vi "Measurement UI.vi"() -> ()   [LabVIEW 2025, in "CAN-LIN Frame Generator UI.lvlib"]
uses:
  CAN-LIN Frame Generator UI.lvlib
  Toggle.ctl
  <vilib>/xnet/xnet.llb/XNET Frame Type CAN.ctl
  OOB gRPC Client/RPC Messages/hwval_GenericRequest.ctl
  OOB gRPC Client/RPC Messages/hwval_BoolRequest.ctl
  <vilib>/Utility/sysdir.llb/System Directory Type.ctl
  OOB gRPC Client/OOB gRPC Client.lvlib
panel:
  in  "HELP":bool
  out "cfg err":bool
  in  "PauseResume":bool caption="Pause"
  out "OOB gRPC Port":i32
  in  "Network":string
  in  "LIN interface":string
  in  "CAN interface":string
  in  "SETTINGS":enum32{"CAN", "LIN"}(tab)
  out "Status CAN":string
  in  "Payload CAN":u32[](array[numeric])=[0, 0, 0, 0, 0, 0, 0, 0, 0, 0, 0, 0, 0, 0, 0, 0, 0, 0, 0, 0, 0, 0, 0, 0, 0, 0, 0, 0, 0, 0, 0, 0, 0, 0, 0, 0, 0, 0, 0, 0, 0, 0, 0, 0, 0, 0, 0, 0, 0, 0, 0, 0, 0, 0, 0, 0, 0, 0, 0, 0, 0, 0, 0, 0] format="%x"
  in  "SEND CAN":bool
  in  "DLC CAN":u32=8
  in  "Type CAN":T1 items=["CAN Data"=0, "CAN Remote"=1, "CAN Bus Error"=2, "CAN 2.0 Data"=8, "CAN FD Data"=16, "CAN FD+BRS Data"=24, "J1939 Data"=192, "Delay"=224, "Log Trigger"=225, "Start Trigger"=226]
  in  "ID CAN":u32 format="%x"
  in  "IO Mode CAN":enum32{"CAN", "CAN FD", "CAN FD + BRS"}(ring)
  in  "FD ISO Mode CAN":enum32{"ISO", "Legacy ISO", "Non-ISO"}(ring)
  in  "Baudrate CAN":u32=125000
  in  "FD Baudrate CAN":u32=1000000
  in  "Termination CAN":T2
  in  "INTERFACE NAME CAN":refnum<k21>
  out "Status LIN":string
  in  "Payload LIN":u32[](array[numeric])=[0, 0, 0, 0, 0, 0, 0, 0] format="%x"
  in  "SEND LIN":bool
  in  "DLC LIN":u32=8
  in  "ID LIN":u32 format="%x"
  in  "Termination LIN":T2
  in  "INTERFACE NAME LIN":refnum<k21>
  in  "Baudrate LIN":u32=19200
  # "CONFIGURATION"
  # "CONTROL"
  # "STATUS"
  # "CONFIGURATION"
  # "CONTROL"
  # "STATUS"
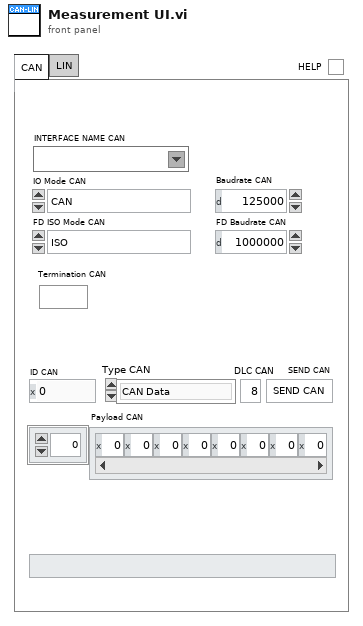
[diagram p1: front panel]
types:
  T1 = typedef "XNET Frame Type CAN.ctl" = u8
  T2 = typedef "Toggle.ctl" = bool
  T3 = enum32{"Page Enabled", "Page Disabled", "Page Disabled & Grayed"}
  T4 = typedef "OOB gRPC Client.lvlib/hwval_GenericRequest.ctl" = cluster{"Command":string, "Payload":u8[]}
  T5 = typedef "OOB gRPC Client.lvlib/hwval_BoolRequest.ctl" = cluster{"BooleanData":bool}
  T6 = enum8{"Enabled", "Disabled", "Disabled and Grayed Out"}
  T7 = typedef "grpc-lvsupport-release.lvlib/grpcId.ctl" = u64
  T8 = typedef "System Directory Type.ctl" = i32
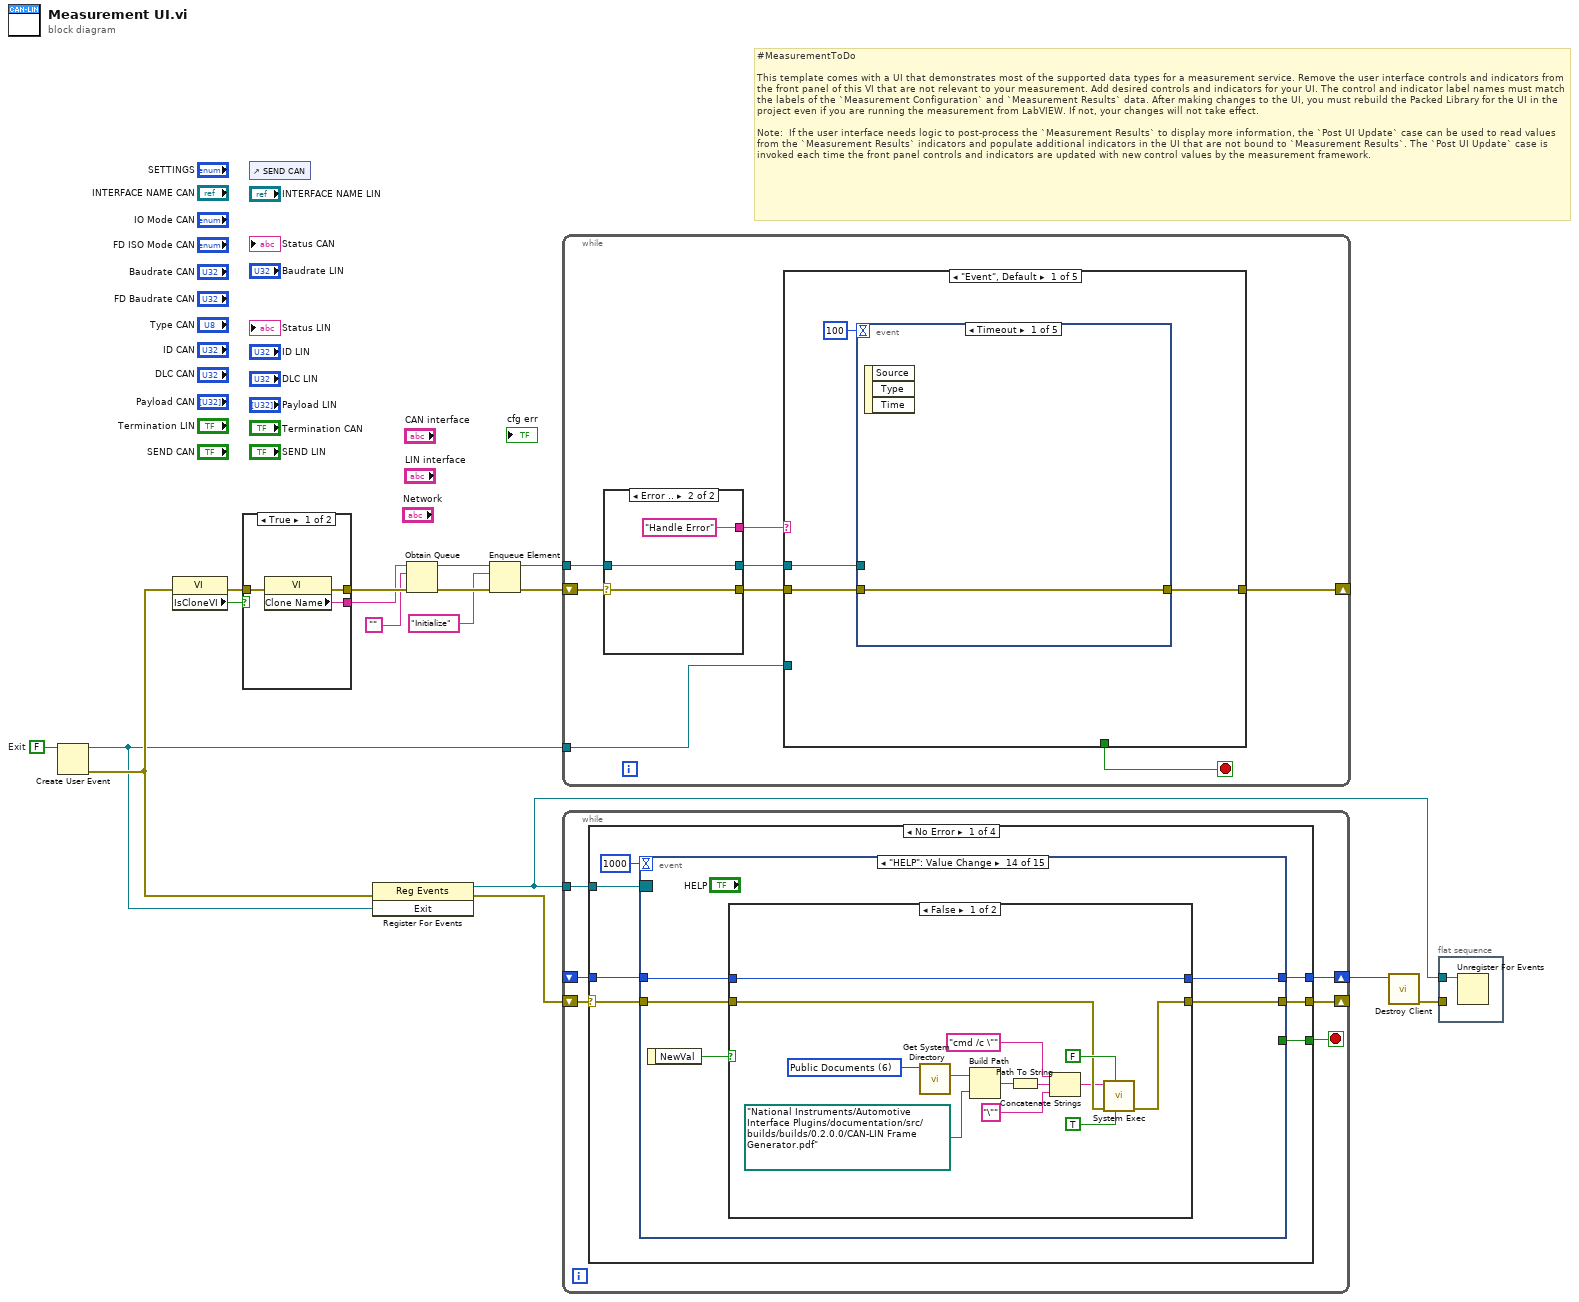
[diagram p0: block diagram]
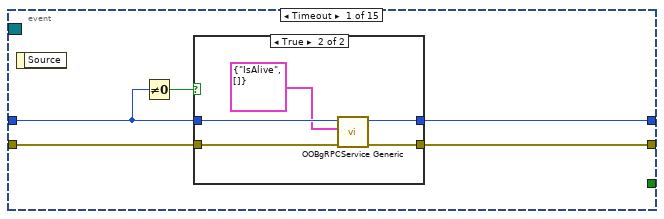
[diagram p2: hidden frame]
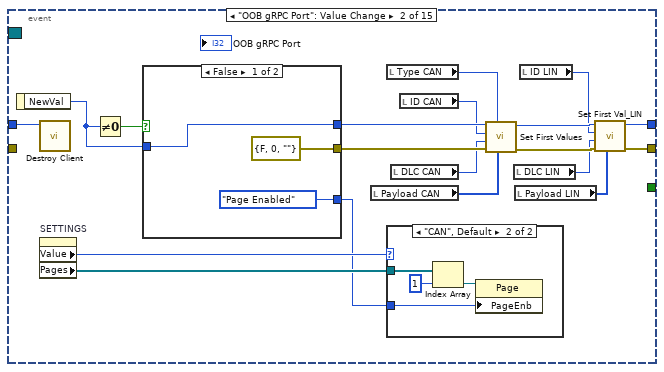
[diagram p4: hidden frame]
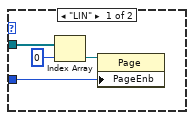
[diagram p5: hidden frame]
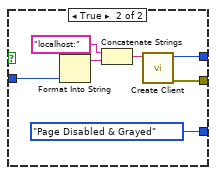
[diagram p6: hidden frame]
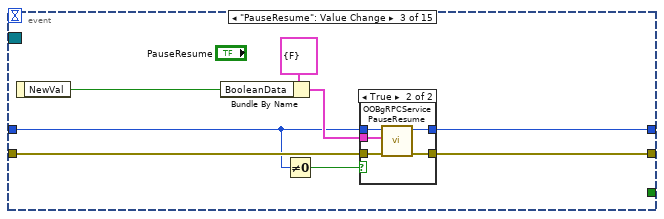
[diagram p7: hidden frame]
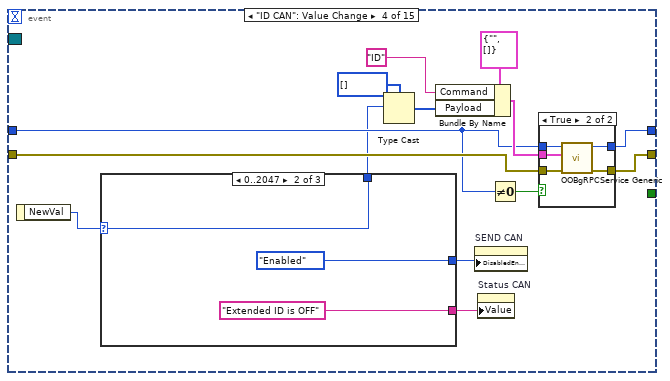
[diagram p9: hidden frame]
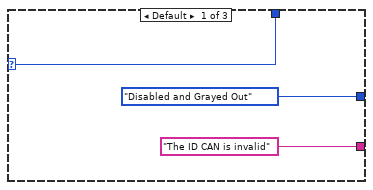
[diagram p10: hidden frame]
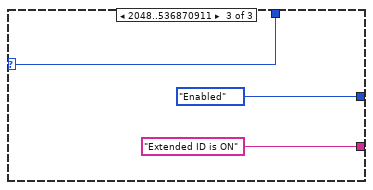
[diagram p11: hidden frame]
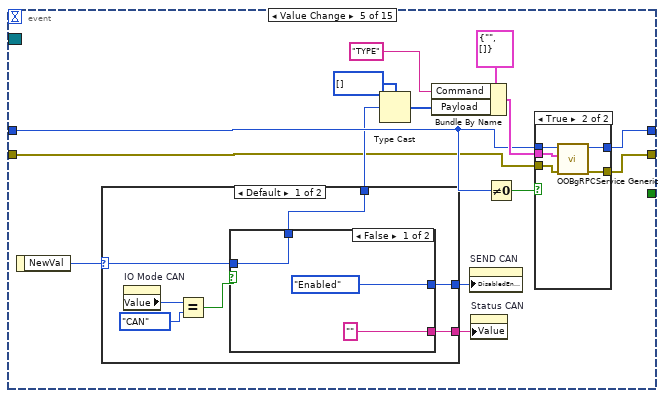
[diagram p13: hidden frame]
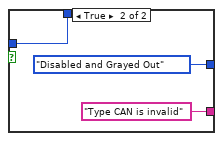
[diagram p14: hidden frame]
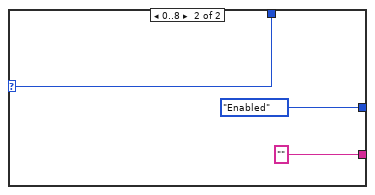
[diagram p15: hidden frame]
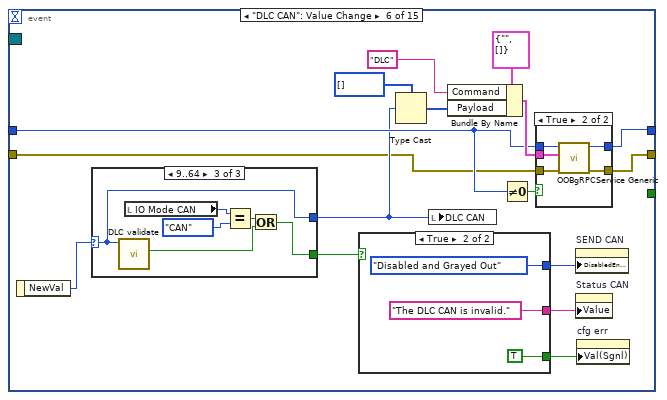
[diagram p17: hidden frame]
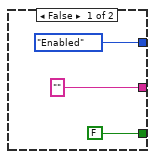
[diagram p18: hidden frame]
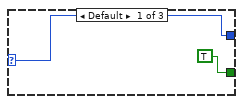
[diagram p19: hidden frame]
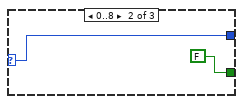
[diagram p20: hidden frame]
diagram:
  w7 = FALSE  # Exit
  # "#MeasurementToDo  \n\nThis template comes with a UI that demonstrates most of the supported data types for a measurement service. Remove the user interface controls and indicators from the front panel of this VI that are not relevant to your measurement. Add desired controls and indicators for your UI. The control and indicator label names must match the labels of the `Measurement Configuration` and `Measurement Results` data. After making changes to the UI, you must rebuild the Packed Library for the UI in the project even if you are running the measurement from LabVIEW. If not, your changes will not take effect.\n\nNote:  If the user interface needs logic to post-process the `Measurement Results` to display more information, the `Post UI Update` case can be used to read values from the `Measurement Results` indicators and populate additional indicators in the UI that are not bound to `Measurement Results`. The `Post UI Update` case is invoked each time the front panel controls and indicators are updated with new control values by the measurement framework."
  n1 = Create User Event(user event datatype=w7) -> (user event=w2:refnum<user-event>, error out=w3:errorcluster)  [unwired: 1 in]
  n2 = property class="VI"(error in=w3) -> (error out=w8:errorcluster, "IsCloneVI"=w9:bool)  [unwired: 1 in, 1 out]
  n3 = case shown="True" w9 {
    tunnel: [w20 w23] -> w17
    tunnel: [w19 w22] -> w16
    tunnel: w8 -> [w18 w21]
    frame True {
      n4 = property class="VI"(error in=w18) -> (error out=w20:errorcluster, "Clone Name"=w19:string)  [unwired: 1 in, 1 out]
    }
    frame False {
      n5 = property class="VI"(error in=w21) -> (error out=w23:errorcluster, "Name"=w22:string)  [unwired: 1 in, 1 out]
    }
  }
  n6 = control-ref of="SEND CAN"() -> ()  [unwired: 1 out]
  n7 = register-events(error in=w3, w2) -> (reference out=w1:refnum<event-registration>, error out=w6:errorcluster)  [unwired: 1 in]
  n8 = Obtain Queue(name (unnamed)=w16, element data type="", error in (no error)=w17) -> (queue out=w13:refnum<queue>, error out=w15:errorcluster)  [unwired: 2 in, 1 out]
  n9 = Enqueue Element(queue=w13, element="Initialize", error in (no error)=w15) -> (queue out=w12:refnum<queue>, error out=w14:errorcluster)  [unwired: 1 in, 1 out]
  n10 = while {
    shift-right: [w26] -> _
    shift-left: w14 -> [w31]
    tunnel: w12 -> [w29]
    tunnel: w2 -> [w24]
    stop <- w25 stop-if-true
    n11 = case shown="Error .." w31 {
      selector: w31 -> [w37 w40]
      tunnel: [w36 w40] -> w30
      tunnel: w29 -> [w35 w39]
      tunnel: [w34 w39] -> w28
      tunnel: [w33 "Handle Error"] -> w27
      frame No Error {
        n12 = Dequeue Element(queue=w35, timeout in ms (-1)=100, error in (no error)=w37) -> (queue out=w34:refnum<queue>, element=w33:string, error out=w36:errorcluster)  [unwired: 1 out]
      }
      frame Error {
      }
    }
    n13 = case shown="\"Event\", Default" w27 {
      tunnel: w30 -> [w43 w61 w70 w83 w84]
      tunnel: w28 -> [w41 _ _ w81 _]
      tunnel: [w44 w61 w70 w72 w84] -> w26
      tunnel: [_ FALSE _ TRUE _] -> w25
      tunnel: w24 -> [_ _ _ w76 _]
      frame "Event", Default {
        n14 = event shown="[0] Timeout" {
          selector: _ -> [_ _ _ _ _]
          dyn-events: _ -> [_ _ _ _ _]
          timeout: 100 -> [_ _ _ _ _]
          tunnel: [w45 w48 _ w52 w54] -> w44
          tunnel: w43 -> [w45 w49 _ w52 w54]
          tunnel: w41 -> [_ w47 _ _ _]
          event Timeout {
            n15 = event-data() -> ()  [unwired: 1 in, 3 out]
          }
          event Panel Close? {
            n16 = event-data() -> ()  [unwired: 1 in, 4 out]
            n17 = Enqueue Element(queue=w47, element="Exit", error in (no error)=w49) -> (error out=w48:errorcluster)  [unwired: 1 in, 2 out]
            n18 = event-data("Discard?"=TRUE) -> ()  [unwired: 1 in, 1 out]
          }
          event "INTERFACE NAME CAN": Value Change {
            n19 = event-data() -> ("NewVal"=w51:refnum<k21>)  [unwired: 1 in, 5 out]
            n20 = property on="CAN interface" class="Str"("Value"=w51) -> ()  [unwired: 2 in, 2 out]
          }
          event "INTERFACE NAME LIN": Value Change {
            n21 = event-data() -> ("NewVal"=w53:refnum<k21>)  [unwired: 1 in, 5 out]
            n22 = property on="LIN interface" class="Str"("Value"=w53) -> ()  [unwired: 2 in, 2 out]
          }
          event "SETTINGS": Value Change {
            n23 = event-data() -> ("NewVal"=w55:enum32{"CAN", "LIN"})  [unwired: 1 in, 5 out]
            n24 = case shown="\"CAN\", Default" w55 {
              frame "CAN", Default {
                n25 = property on="Network" class="Str"("Value"="CAN" ("Tab No")) -> ()  [unwired: 2 in, 2 out]
              }
              frame "LIN" {
                n26 = property on="Network" class="Str"("Value"="LIN" ("Tab No")) -> ()  [unwired: 2 in, 2 out]
              }
            }
          }
        }
      }
      frame "Initialize" {
        n27 = property on="SETTINGS" class="TabCtl (strict)"() -> ("Pages"=w58:refnum<vi>[])  [unwired: 2 in, 2 out]
        n28 = for {
          tunnel: w58 -> [w63] mode=indexing
          n29 = property class="Page"(reference=w63, "PageEnb"=T3."Page Enabled" ("Page Enabled State")) -> ()  [unwired: 1 in, 2 out]
        }
        n30 = property on="Network" class="Str"("Value"="CAN" ("Tab No")) -> ()  [unwired: 2 in, 2 out]
      }
      frame "Post UI Update" {
        # "Generate an event when grpc port value is not equal to 0 and it has changed."
        # "This case will be triggered, after framework updates the User interface with result values."
        n31 = local read "OOB gRPC Port"() -> (w65:i32)
        n32 = feedback #1(0 ("OOB gRPC Port")) -> (w64:i32)
        n33 = feedback-in #1(w65) -> ()
        n34 = Not Equal?(x=w65, y=w64) -> (x != y?=w66:bool)
        n35 = Not Equal To 0?(x=w65) -> (x != 0?=w68:bool)
        n36 = Compound Arithmetic op=AND(w68, w66) -> (w67:bool)
        n37 = case shown="True" w67 {
          tunnel: w65 -> [_ w71]
          frame False {
          }
          frame True {
            n38 = property on="OOB gRPC Port" class="DigNum (strict)"("Val(Sgnl)"=w71) -> ()  [unwired: 2 in, 2 out]
          }
        }
      }
      frame "Exit" {
        # "This case is triggered to close the User Interface from framework"
        n39 = Generate User Event(user event=w76, event data cluster=TRUE) -> (user event out=w77:refnum<user-event>)  [unwired: 2 in, 1 out]
        n40 = Flush Queue(queue=w81, error in (no error)=w83) -> (queue out=w80:refnum<queue>, error out=w79:errorcluster)  [unwired: 1 out]
        n41 = Destroy User Event(user event=w77) -> (error out=w73:errorcluster)  [unwired: 1 in]
        n42 = Release Queue(queue=w80, force destroy? (F)=TRUE, error in (no error)=w79) -> (error out=w74:errorcluster)  [unwired: 2 out]
        n43 = Merge Errors(w74, w73) -> (w72:errorcluster)
      }
      frame "Handle Error" {
      }
    }
  }
  n44 = while {
    tunnel: w1 -> [w87]
    shift-right: [w88] -> _
    shift-left: w6 -> [w90]
    shift-right: [w85] -> w4
    shift-left: _ -> [w86]
    stop <- w89 stop-if-true
    n45 = case shown="No Error" w90 {
      selector: w90 -> [w95 w435 _ _]
      tunnel: [w92 TRUE w440 w446] -> w89
      tunnel: [w96 w435 errorcluster {"status"=FALSE, "code"=0, "source"=""} ("error IO") errorcluster {"status"=FALSE, "code"=0, "source"=""} ("error IO")] -> w88
      tunnel: w87 -> [w97 _ _ _]
      tunnel: w86 -> [w94 w436 w439 w445]
      tunnel: [w93 w436 w439 w445] -> w85
      frame No Error {
        n46 = event shown="[13] \"HELP\": Value Change" {
          selector: w97 -> [_ _ _ _ _ _ _ _ _ _ _ _ _ _ _]
          dyn-events: _ -> [_ _ _ _ _ _ _ _ _ _ _ _ _ _ _]
          timeout: 1000 -> [_ _ _ _ _ _ _ _ _ _ _ _ _ _ _]
          tunnel: [w100 w118 w153 w168 w197 w237 w268 w290 w317 w340 w359 w377 w394 w415 w432] -> w96
          tunnel: w95 -> [w101 _ w152 w171 w194 w233 w271 w293 w319 w343 w361 w385 w397 w414 w432]
          tunnel: w94 -> [w99 w128 w147 w166 w199 w236 w272 w292 w320 w342 w360 w384 w396 w413 w433]
          tunnel: [w102 w119 w154 w169 w198 w238 w269 w291 w318 w341 w358 w376 w395 w412 w433] -> w93
          tunnel: [_ _ _ _ _ _ _ _ _ _ _ _ _ _ w434] -> w92
          event Timeout {
            n47 = event-data() -> ()  [unwired: 1 in, 1 out]
            n48 = Not Equal To 0?(x=w99) -> (x != 0?=w98:bool)
            n49 = case shown="True" w98 {
              tunnel: w99 -> [w104 w108]
              tunnel: [w104 w109] -> w102
              tunnel: w101 -> [w103 w106]
              tunnel: [w103 w107] -> w100
              frame False {
              }
              frame True {
                n50 = call "OOBgRPCService Generic.vi"("error in"=w106, "Request Data"=T4 {"Command"="IsAlive", "Payload"=[]}, "gRPC ID"=w108) -> ("error out"=w107:errorcluster, "gRPC ID out"=w109:T7)  [unwired: 6 in, 1 out]
              }
            }
          }
          event "OOB gRPC Port": Value Change {
            n51 = event-data() -> ("NewVal"=w126:i32)  [unwired: 1 in]
            n52 = call "Destroy Client.vi"("gRPC ID"=w128) -> ()  [unwired: 10 in, 1 out]
            n53 = property on="SETTINGS" class="TabCtl (strict)"() -> ("Value"=w111:enum32{"CAN", "LIN"}, "Pages"=w112:refnum<vi>[])  [unwired: 2 in, 2 out]
            n54 = Not Equal To 0?(x=w126) -> (x != 0?=w127:bool)
            n55 = case shown="False" w127 {
              tunnel: [errorcluster {"status"=FALSE, "code"=0, "source"=""} ("error out") w146] -> w124
              tunnel: w126 -> [w139 w142]
              tunnel: [w139 w141] -> w125
              tunnel: [T3."Page Enabled" ("Page Enabled State") T3."Page Disabled & Grayed" ("Page Enabled State")] -> w110
              frame False {
              }
              frame True {
                n56 = Format Into String(w142) -> (resulting string=w145:string)  [unwired: 3 in, 1 out]
                n57 = Concatenate Strings("localhost:" ("string"), w145) -> (w143:string)
                n58 = call "Create Client.vi"("address"=w143) -> ("error out"=w146:errorcluster, "gRPC ID Out"=w141:T7)  [unwired: 9 in]
              }
            }
            n59 = local read "Payload CAN"() -> (w120:u32[])
            n60 = local read "Type CAN"() -> (w121:T1)
            n61 = case shown="\"CAN\", Default" w111 {
              tunnel: w112 -> [w130 w134]
              tunnel: w110 -> [w129 w133]
              frame "LIN" {
                n62 = Index Array(array=w130, index=0) -> (element=w132:refnum<vi>)
                n63 = property class="Page"(reference=w132, "PageEnb"=w129) -> ()  [unwired: 1 in, 2 out]
              }
              frame "CAN", Default {
                n64 = Index Array(array=w134, index=1) -> (element=w136:refnum<vi>)
                n65 = property class="Page"(reference=w136, "PageEnb"=w133) -> ()  [unwired: 1 in, 2 out]
              }
            }
            n66 = local read "DLC CAN"() -> (w122:u32)
            n67 = local read "ID CAN"() -> (w123:u32)
            n68 = call "Set First Values.vi"("PAYLOAD"=w120, "TYPE"=w121, "error"=w124, "DLC"=w122, "IDENTIFIER"=w123, "gRPC ID In"=w125) -> ("error out"=w116:errorcluster, "gRPC ID Out"=w117:T7)  [unwired: 4 in]
            n69 = local read "DLC LIN"() -> (w114:u32)
            n70 = local read "Payload LIN"() -> (w115:u32[])
            n71 = local read "ID LIN"() -> (w113:u32)
            n72 = call "Set First Val_LIN.vi"("Payload LIN"=w115, "error in"=w116, "DLC LIN"=w114, "ID LIN"=w113, "gRPC ID"=w117) -> ("error out"=w118:errorcluster, "gRPC ID out"=w119:T7)  [unwired: 5 in]
          }
          event "PauseResume": Value Change {
            n73 = event-data() -> ("NewVal"=w149:bool)  [unwired: 1 in]
            n74 = Bundle By Name(cluster=T5 {"BooleanData"=FALSE} ("Request Data"), "BooleanData"=w149) -> (w150:T5)
            n75 = Not Equal To 0?(x=w147) -> (x != 0?=w148:bool)
            n76 = case shown="True" w148 {
              tunnel: [w156 w161] -> w154
              tunnel: [w155 w160] -> w153
              tunnel: w147 -> [w156 w159]
              tunnel: w152 -> [w155 w158]
              tunnel: w150 -> [_ w157]
              frame False {
              }
              frame True {
                n77 = call "OOBgRPCService PauseResume.vi"("error in"=w158, "Request Data"=w157, "gRPC ID"=w159) -> ("error out"=w160:errorcluster, "gRPC ID out"=w161:T7)  [unwired: 6 in, 1 out]
              }
            }
          }
          event "ID CAN": Value Change {
            n78 = event-data() -> ("NewVal"=w165:u32)  [unwired: 1 in]
            n79 = case shown="0..2047" w165 {
              selector: w165 -> [w178 w181 w184]
              tunnel: [w178 w181 w184] -> w164
              tunnel: [T6."Disabled and Grayed Out" ("Disabled") T6."Enabled" ("Disabled") T6."Enabled" ("Disabled")] -> w163
              tunnel: ["The ID CAN is invalid" ("Status LIN") "Extended ID is OFF" ("Status LIN") "Extended ID is ON" ("Status LIN")] -> w162
              frame Default {
              }
              frame 0..2047 {
              }
              frame 2048..536870911 {
              }
            }
            n80 = Type Cast(type=u8[] [] ("Payload"), x=w164) -> (*(type *) &x=w172:u8[])
            n81 = Bundle By Name(cluster=T4 {"Command"="", "Payload"=[]} ("hwval_GenericRequest"), "Command"="ID", "Payload"=w172) -> (w170:T4)
            n82 = property on="SEND CAN" class="Bool (strict)"("DisabledEnum"=w163) -> ()  [unwired: 2 in, 2 out]
            n83 = property on="Status CAN" class="Str"("Value"=w162) -> ()  [unwired: 2 in, 2 out]
            n84 = Not Equal To 0?(x=w166) -> (x != 0?=w167:bool)
            n85 = case shown="True" w167 {
              tunnel: [w186 w188] -> w169
              tunnel: [w185 w187] -> w168
              tunnel: w166 -> [w186 w191]
              tunnel: w171 -> [w185 w190]
              tunnel: w170 -> [_ w189]
              frame False {
              }
              frame True {
                n86 = call "OOBgRPCService Generic.vi"("error in"=w190, "Request Data"=w189, "gRPC ID"=w191) -> ("error out"=w187:errorcluster, "gRPC ID out"=w188:T7)  [unwired: 6 in, 1 out]
              }
            }
          }
          event Value Change {
            n87 = event-data() -> ("NewVal"=w196:T1)  [unwired: 1 in]
            n88 = case shown="Default" w196 {
              selector: w196 -> [w209 w221]
              tunnel: [w208 w221] -> w195
              tunnel: [w207 T6."Enabled" ("Disabled")] -> w193
              tunnel: [w206 "" ("Status CAN")] -> w192
              frame Default {
                n89 = property on="IO Mode CAN" class="Enum (strict)"() -> ("Value"=w212:enum32{"CAN", "CAN FD", "CAN FD + BRS"})  [unwired: 2 in, 2 out]
                n90 = Equal?(x=w212, y=enum32{"CAN", "CAN FD", "CAN FD + BRS"}."CAN") -> (x = y?=w210:bool)
                n91 = case shown="False" w210 {
                  tunnel: w209 -> [w213 w216]
                  tunnel: [w213 w216] -> w208
                  tunnel: [T6."Enabled" ("Disabled") T6."Disabled and Grayed Out" ("Disabled")] -> w207
                  tunnel: ["" ("Status CAN") "Type CAN is invalid" ("Status CAN")] -> w206
                  frame False {
                  }
                  frame True {
                  }
                }
              }
              frame 0..8 {
              }
            }
            n92 = Type Cast(type=u8[] [] ("Payload"), x=w195) -> (*(type *) &x=w202:u8[])
            n93 = Bundle By Name(cluster=T4 {"Command"="", "Payload"=[]} ("hwval_GenericRequest"), "Command"="TYPE", "Payload"=w202) -> (w201:T4)
            n94 = property on="SEND CAN" class="Bool (strict)"("DisabledEnum"=w193) -> ()  [unwired: 2 in, 2 out]
            n95 = property on="Status CAN" class="Str"("Value"=w192) -> ()  [unwired: 2 in, 2 out]
            n96 = Not Equal To 0?(x=w199) -> (x != 0?=w200:bool)
            n97 = case shown="True" w200 {
              tunnel: [w223 w225] -> w198
              tunnel: [w222 w224] -> w197
              tunnel: w199 -> [w223 w228]
              tunnel: w194 -> [w222 w227]
              tunnel: w201 -> [_ w226]
              frame False {
              }
              frame True {
                n98 = call "OOBgRPCService Generic.vi"("error in"=w227, "Request Data"=w226, "gRPC ID"=w228) -> ("error out"=w224:errorcluster, "gRPC ID out"=w225:T7)  [unwired: 6 in, 1 out]
              }
            }
          }
          event "DLC CAN": Value Change {
            n99 = event-data() -> ("NewVal"=w235:u32)  [unwired: 1 in]
            n100 = case shown="9..64" w235 {
              selector: w235 -> [w252 w254 w255]
              tunnel: [w252 w254 w255] -> w234
              tunnel: [TRUE FALSE w256] -> w232
              frame Default {
              }
              frame 0..8 {
              }
              frame 9..64 {
                n101 = call "DLC validate.vi"("in"=w255) -> ("invalid?"=w257:bool)  [unwired: 8 in, 2 out]
                n102 = local read "IO Mode CAN"() -> (w260:enum32{"CAN", "CAN FD", "CAN FD + BRS"})
                n103 = Equal?(x=w260, y=enum32{"CAN", "CAN FD", "CAN FD + BRS"}."CAN") -> (x = y?=w258:bool)
                n104 = Or(x=w258, y=w257) -> (x .or. y?=w256:bool)
              }
            }
            n105 = case shown="True" w232 {
              tunnel: ["" ("Status CAN") "The DLC CAN is invalid." ("Status CAN")] -> w231
              tunnel: [T6."Enabled" ("Disabled") T6."Disabled and Grayed Out" ("Disabled")] -> w230
              tunnel: [FALSE ("Value (Signaling)") TRUE ("Value (Signaling)")] -> w229
              frame False {
              }
              frame True {
              }
            }
            n106 = Type Cast(type=u8[] [] ("Payload"), x=w234) -> (*(type *) &x=w241:u8[])
            n107 = local write "DLC CAN"(w234) -> ()
            n108 = Bundle By Name(cluster=T4 {"Command"="", "Payload"=[]} ("hwval_GenericRequest"), "Command"="DLC", "Payload"=w241) -> (w240:T4)
            n109 = Not Equal To 0?(x=w236) -> (x != 0?=w239:bool)
            n110 = case shown="True" w239 {
              tunnel: [w262 w264] -> w238
              tunnel: [w261 w263] -> w237
              tunnel: w236 -> [w262 w267]
              tunnel: w233 -> [w261 w266]
              tunnel: w240 -> [_ w265]
              frame False {
              }
              frame True {
                n111 = call "OOBgRPCService Generic.vi"("error in"=w266, "Request Data"=w265, "gRPC ID"=w267) -> ("error out"=w263:errorcluster, "gRPC ID out"=w264:T7)  [unwired: 6 in, 1 out]
              }
            }
            n112 = property on="SEND CAN" class="Bool (strict)"("DisabledEnum"=w230) -> ()  [unwired: 2 in, 2 out]
            n113 = property on="Status CAN" class="Str"("Value"=w231) -> ()  [unwired: 2 in, 2 out]
            n114 = property on="cfg err" class="Bool (strict)"("Val(Sgnl)"=w229) -> ()  [unwired: 2 in, 2 out]
          }
          event "Payload CAN": Value Change {
            n115 = event-data() -> ("NewVal"=w270:u32[])  [unwired: 1 in]
            n116 = Type Cast(type=u8[] [] ("Payload"), x=w270) -> (*(type *) &x=w275:u8[])
            n117 = Bundle By Name(cluster=T4 {"Command"="", "Payload"=[]} ("hwval_GenericRequest"), "Command"="PAYLOAD", "Payload"=w275) -> (w274:T4)
            n118 = Not Equal To 0?(x=w272) -> (x != 0?=w273:bool)
            n119 = case shown="True" w273 {
              tunnel: [w280 w282] -> w269
              tunnel: [w279 w281] -> w268
              tunnel: w272 -> [w280 w285]
              tunnel: w271 -> [w279 w284]
              tunnel: w274 -> [_ w283]
              frame False {
              }
              frame True {
                n120 = call "OOBgRPCService Generic.vi"("error in"=w284, "Request Data"=w283, "gRPC ID"=w285) -> ("error out"=w281:errorcluster, "gRPC ID out"=w282:T7)  [unwired: 6 in, 1 out]
              }
            }
          }
          event "ID LIN": Value Change {
            n121 = event-data() -> ("NewVal"=w289:u32)  [unwired: 1 in]
            n122 = case shown="Default" w289 {
              selector: w289 -> [w302 w305]
              tunnel: [w302 w305] -> w288
              tunnel: [T6."Disabled and Grayed Out" ("Disabled") T6."Enabled" ("Disabled")] -> w287
              tunnel: ["The maximum value of ID LIN is 0x3F" ("Status LIN") "" ("Status LIN")] -> w286
              frame Default {
              }
              frame 0..63 {
              }
            }
            n123 = Type Cast(type=u8[] [] ("Payload"), x=w288) -> (*(type *) &x=w296:u8[])
            n124 = property on="SEND LIN" class="Bool (strict)"("DisabledEnum"=w287) -> ()  [unwired: 2 in, 2 out]
            n125 = property on="Status LIN" class="Str"("Value"=w286) -> ()  [unwired: 2 in, 2 out]
            n126 = Bundle By Name(cluster=T4 {"Command"="", "Payload"=[]} ("hwval_GenericRequest"), "Command"="ID2", "Payload"=w296) -> (w295:T4)
            n127 = Not Equal To 0?(x=w292) -> (x != 0?=w294:bool)
            n128 = case shown="True" w294 {
              tunnel: [w307 w309] -> w291
              tunnel: [w306 w308] -> w290
              tunnel: w292 -> [w307 w312]
              tunnel: w293 -> [w306 w311]
              tunnel: w295 -> [_ w310]
              frame False {
              }
              frame True {
                n129 = call "OOBgRPCService Generic.vi"("error in"=w311, "Request Data"=w310, "gRPC ID"=w312) -> ("error out"=w308:errorcluster, "gRPC ID out"=w309:T7)  [unwired: 6 in, 1 out]
              }
            }
          }
          event "DLC LIN": Value Change {
            n130 = event-data() -> ("NewVal"=w316:u32)  [unwired: 1 in]
            n131 = case shown="Default" w316 {
              selector: w316 -> [w329 w332]
              tunnel: [w329 w332] -> w315
              tunnel: [T6."Disabled and Grayed Out" ("Disabled") T6."Enabled" ("Disabled")] -> w314
              tunnel: ["The DLC LIN is invalid." ("Status CAN") "" ("Status CAN")] -> w313
              frame Default {
              }
              frame 0..8 {
              }
            }
            n132 = property on="SEND LIN" class="Bool (strict)"("DisabledEnum"=w314) -> ()  [unwired: 2 in, 2 out]
            n133 = Type Cast(type=u8[] [] ("Payload"), x=w315) -> (*(type *) &x=w323:u8[])
            n134 = property on="Status LIN" class="Str"("Value"=w313) -> ()  [unwired: 2 in, 2 out]
            n135 = local write "DLC LIN"(w315) -> ()
            n136 = Bundle By Name(cluster=T4 {"Command"="", "Payload"=[]} ("hwval_GenericRequest"), "Command"="DLC2", "Payload"=w323) -> (w322:T4)
            n137 = Not Equal To 0?(x=w320) -> (x != 0?=w321:bool)
            n138 = case shown="True" w321 {
              tunnel: [w334 w336] -> w318
              tunnel: [w333 w335] -> w317
              tunnel: w320 -> [w334 w339]
              tunnel: w319 -> [w333 w338]
              tunnel: w322 -> [_ w337]
              frame False {
              }
              frame True {
                n139 = call "OOBgRPCService Generic.vi"("error in"=w338, "Request Data"=w337, "gRPC ID"=w339) -> ("error out"=w335:errorcluster, "gRPC ID out"=w336:T7)  [unwired: 6 in, 1 out]
              }
            }
          }
          event "Payload LIN": Value Change {
            n140 = event-data() -> ("NewVal"=w344:u32[])  [unwired: 1 in]
            n141 = Type Cast(type=u8[] [] ("Payload"), x=w344) -> (*(type *) &x=w347:u8[])
            n142 = Bundle By Name(cluster=T4 {"Command"="", "Payload"=[]} ("hwval_GenericRequest"), "Command"="PAYLOAD2", "Payload"=w347) -> (w346:T4)
            n143 = Not Equal To 0?(x=w342) -> (x != 0?=w345:bool)
            n144 = case shown="True" w345 {
              tunnel: [w352 w354] -> w341
              tunnel: [w351 w353] -> w340
              tunnel: w342 -> [w352 w357]
              tunnel: w343 -> [w351 w356]
              tunnel: w346 -> [_ w355]
              frame False {
              }
              frame True {
                n145 = call "OOBgRPCService Generic.vi"("error in"=w356, "Request Data"=w355, "gRPC ID"=w357) -> ("error out"=w353:errorcluster, "gRPC ID out"=w354:T7)  [unwired: 6 in, 1 out]
              }
            }
          }
          event "cfg err": Value Change {
            n146 = event-data() -> ("NewVal"=w362:bool)  [unwired: 1 in]
            n147 = Type Cast(type=u8[] [] ("Payload"), x=w362) -> (*(type *) &x=w365:u8[])
            n148 = Bundle By Name(cluster=T4 {"Command"="", "Payload"=[]} ("hwval_GenericRequest"), "Command"="cfg err", "Payload"=w365) -> (w364:T4)
            n149 = Not Equal To 0?(x=w360) -> (x != 0?=w363:bool)
            n150 = case shown="True" w363 {
              tunnel: [w370 w372] -> w358
              tunnel: [w369 w371] -> w359
              tunnel: w360 -> [w370 w375]
              tunnel: w361 -> [w369 w374]
              tunnel: w364 -> [_ w373]
              frame False {
              }
              frame True {
                n151 = call "OOBgRPCService Generic.vi"("error in"=w374, "Request Data"=w373, "gRPC ID"=w375) -> ("error out"=w371:errorcluster, "gRPC ID out"=w372:T7)  [unwired: 6 in, 1 out]
              }
            }
          }
          event "SEND CAN": Value Change {
            n152 = event-data() -> ("NewVal"=w380:bool)  [unwired: 1 in]
            n153 = Type Cast(type=u8[] [] ("Payload"), x=w380) -> (*(type *) &x=w381:u8[])
            n154 = Bundle By Name(cluster=T4 {"Command"="", "Payload"=[]} ("hwval_GenericRequest"), "Command"="SEND", "Payload"=w381) -> (w378:T4)
            n155 = Not Equal To 0?(x=w384) -> (x != 0?=w386:bool)
            n156 = case shown="True" w386 {
              tunnel: [w388 w390] -> w376
              tunnel: [w387 w389] -> w377
              tunnel: w384 -> [w388 w393]
              tunnel: w385 -> [w387 w392]
              tunnel: w378 -> [_ w391]
              frame False {
              }
              frame True {
                n157 = call "OOBgRPCService Generic.vi"("error in"=w392, "Request Data"=w391, "gRPC ID"=w393) -> ("error out"=w389:errorcluster, "gRPC ID out"=w390:T7)  [unwired: 6 in, 1 out]
              }
            }
          }
          event "SEND LIN": Value Change {
            n158 = event-data() -> ("NewVal"=w398:bool)  [unwired: 1 in]
            n159 = Type Cast(type=u8[] [] ("Payload"), x=w398) -> (*(type *) &x=w401:u8[])
            n160 = Bundle By Name(cluster=T4 {"Command"="", "Payload"=[]} ("hwval_GenericRequest"), "Command"="SEND2", "Payload"=w401) -> (w399:T4)
            n161 = Not Equal To 0?(x=w396) -> (x != 0?=w404:bool)
            n162 = case shown="True" w404 {
              tunnel: [w406 w408] -> w395
              tunnel: [w405 w407] -> w394
              tunnel: w396 -> [w406 w411]
              tunnel: w397 -> [w405 w410]
              tunnel: w399 -> [_ w409]
              frame False {
              }
              frame True {
                n163 = call "OOBgRPCService Generic.vi"("error in"=w410, "Request Data"=w409, "gRPC ID"=w411) -> ("error out"=w407:errorcluster, "gRPC ID out"=w408:T7)  [unwired: 6 in, 1 out]
              }
            }
          }
          event "HELP": Value Change {
            n164 = event-data() -> ("NewVal"=w416:bool)  [unwired: 1 in]
            n165 = case shown="False" w416 {
              tunnel: [w417 w431] -> w415
              tunnel: w414 -> [w419 w431]
              tunnel: w413 -> [w429 w430]
              tunnel: [w429 w430] -> w412
              frame False {
                w428 = T8 6 items=["User Home"=0, "User Desktop"=1, "User Documents"=2, "User Application Data"=3, "User Preferences"=4, "User Temporary"=5, "Public Documents"=6, "Public Application Data"=7, "Public Preferences"=8, "Public Cache"=13, "System Core Libraries"=9, "System Installed Libraries"=10, "Application Files"=11, "Boot Volume Root"=12] ("system directory type")
                n166 = call <vilib>:"Get System Directory.vi"("system directory type"=w428) -> ("system directory"=w427:path)  [unwired: 10 in]
                n167 = Build Path(base path=w427, name or relative path=path "National Instruments/Automotive Interface Plugins/documentation/src/builds/builds/0.2.0.0/CAN-LIN Frame Generator.pdf") -> (appended path=w425:path)
                n168 = Path To String(path=w425) -> (string=w423:string)
                n169 = Concatenate Strings("cmd /c \"", w423, "\"") -> (w418:string)
                n170 = call <vilib>:"System Exec.vi"("run minimized? (F)"=TRUE, "wait until completion? (T)"=FALSE, "error in (no error)"=w419, "command line"=w418) -> ("error out"=w417:errorcluster)  [unwired: 4 in, 3 out]
              }
              frame True {
              }
            }
          }
          event User Event {
            n171 = event-data() -> ("Exit"=w434:bool)  [unwired: 1 in]
          }
        }
      }
      frame Default {
      }
      frame Error {
        n172 = local read "OOB gRPC Port"() -> (w442:i32)
        n173 = Equal?(x=w442, y=-1 ("x")) -> (x = y?=w440:bool)
        n174 = case shown="False" w440 {
          tunnel: w442 -> [w443 _]
          frame False {
            # "triggers event"
            n175 = property on="OOB gRPC Port" class="DigNum (strict)"("Val(Sgnl)"=w443) -> ()  [unwired: 2 in, 2 out]
          }
          frame True {
          }
        }
      }
      frame Error {
        n176 = local read "OOB gRPC Port"() -> (w448:i32)
        n177 = Equal?(x=w448, y=-1 ("x")) -> (x = y?=w446:bool)
        n178 = case shown="False" w446 {
          tunnel: w448 -> [_ _]
          frame False {
            n179 = property on="OOB gRPC Port" class="DigNum (strict)"("Val(Sgnl)"=0 ("Value (Signaling)")) -> ()  [unwired: 2 in, 2 out]
          }
          frame True {
          }
        }
      }
    }
  }
  n180 = call "Destroy Client.vi"("gRPC ID"=w4) -> ("error out"=w5:errorcluster)  [unwired: 10 in]
  n181 = flat-sequence {
    tunnel: w1 -> [w450]
    tunnel: w5 -> [_]
    frame #0 {
      n182 = Unregister For Events(event registration refnum=w450) -> ()  [unwired: 1 in, 1 out]
    }
  }
